vi "GetName.vi"(6 "error in":errorcluster, 9 "Structure in":refnum<class "Structure.lvclass">) -> (0 "error out":errorcluster, 3 "Structure out":refnum<class "Structure.lvclass">, 4 "name":string, 5 "UID":string)   [LabVIEW 2014, in "Structure.lvclass"]
uses:
  Structure.lvclass
  Python/Parsing/Python Functions.lvlib
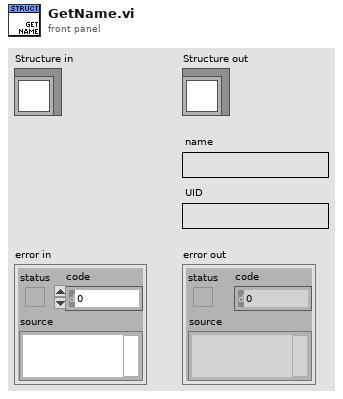
[diagram p1: front panel]
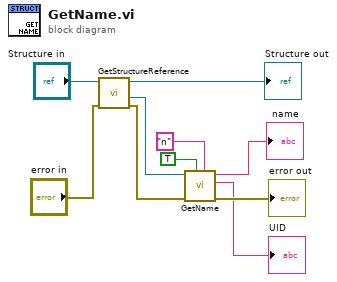
[diagram p0: block diagram]
diagram:
  n1 = call "GetStructureReference.vi"("error in"="error in", "Structure in"="Structure in") -> ("error out"=w10:errorcluster, "reference out"=w9:refnum<vi>, "Structure out"=→"Structure out":refnum<class "Structure.lvclass">)  [unwired: 7 in]
  n2 = call "GetName.vi"("base name"="n", "add self"=TRUE, "error in"=w10, "GObj Refnum"=w9) -> ("error out"=→"error out":errorcluster, "UID"=→"UID":string, "name"=→"name":string)  [unwired: 5 in]
